vi "file_io_vi.vi"() -> ()   [LabVIEW 2017]
panel:
  out "letter count":dbl
  out "word count":dbl
  out "j":i32
  out "Array":string[](array[string])
  out "i":i32
  in  "delimiters":string[](array[string])
  out "result array":string[][](array[string])
  in  "format string":string
  in  "array type":string[][](array[string])
  out "text read from file":string
  out "error from read file":errorcluster
  in  "file path (read file)":path
  out "error from write file":errorcluster
  in  "text will be written to file":string
  in  "file path (write file)":path
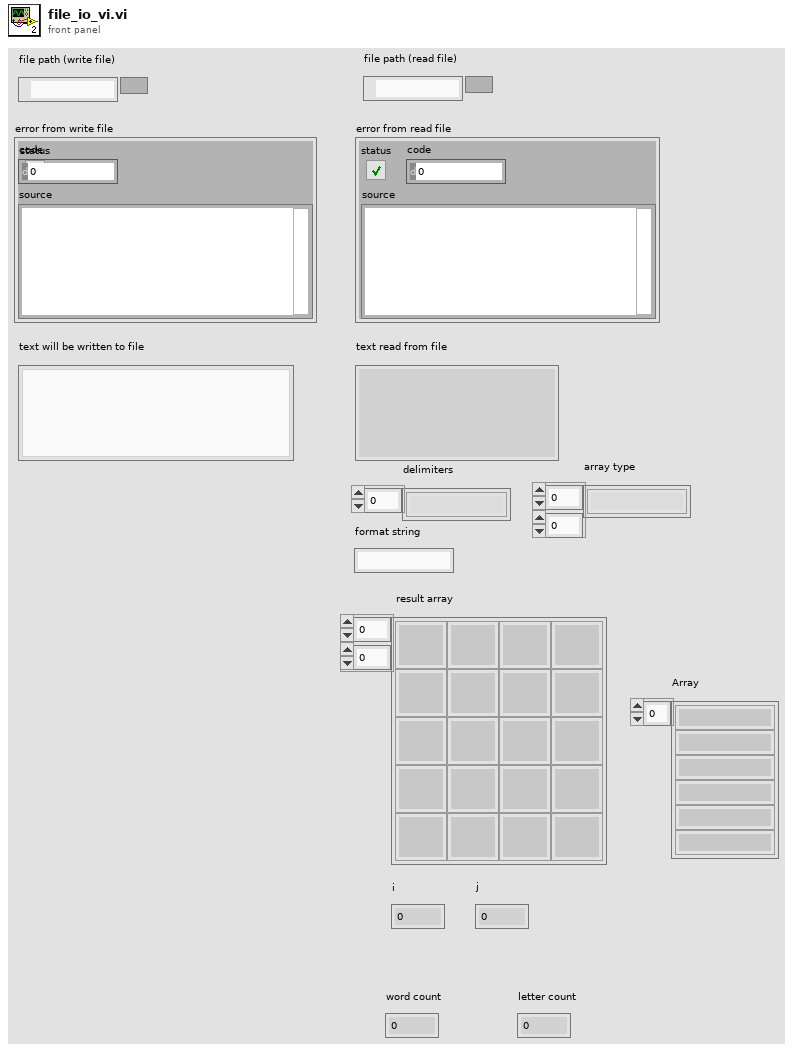
[diagram p1: front panel]
types:
  T1 = enum16{"open", "replace", "create", "open or create", "replace or create", "replace or create with confirmation"}
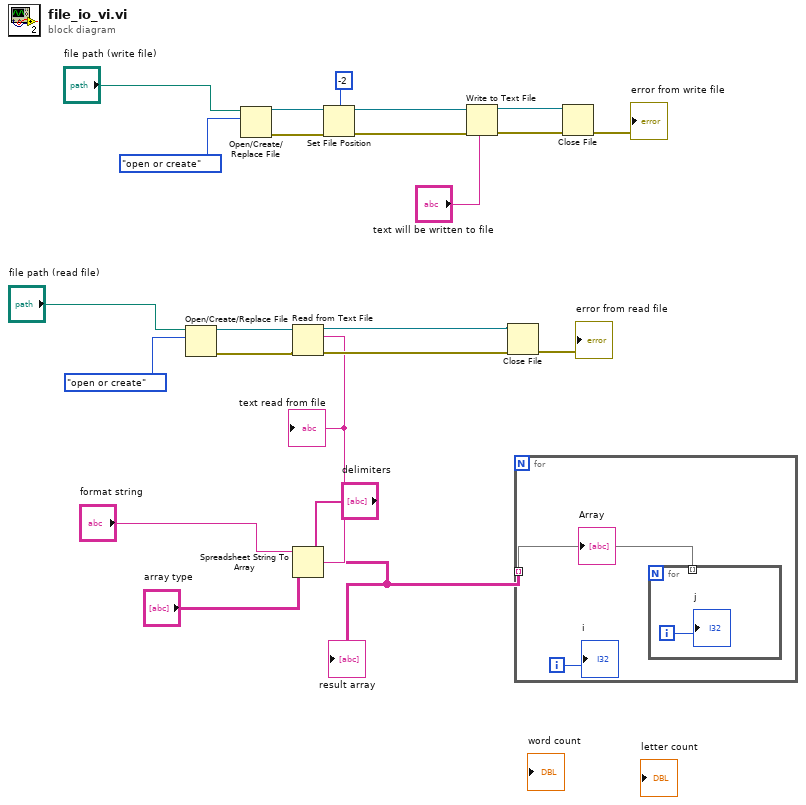
[diagram p0: block diagram]
diagram:
  n1 = Open/Create/Replace File(file path (use dialog)="file path (read file)", operation (0:open)=T1."open or create") -> (refnum out=w9:refnum<file>, error out=w7:errorcluster)  [unwired: 4 in, 1 out]
  n2 = Open/Create/Replace File(file path (use dialog)="file path (write file)", operation (0:open)=T1."open or create") -> (refnum out=w18:refnum<file>, error out=w15:errorcluster)  [unwired: 4 in, 1 out]
  n3 = Read from Text File(file (use dialog)=w9, error in=w7) -> (refnum out=w8:refnum<file>, text=w3:string, error out=w6:errorcluster)  [unwired: 2 in, 1 out]
  "text read from file" <- w3
  n4 = Spreadsheet String To Array(delimiter (Tab)="delimiters", format string="format string", spreadsheet string=w3, array type (2D Dbl)="array type") -> (array=w1:string[][])
  "result array" <- w1
  n5 = Set File Position(offset (in bytes) (0)=i64 -2, refnum=w18, error in=w15) -> (refnum out=w19:refnum<file>, error out=w14:errorcluster)  [unwired: 1 in]
  n6 = Write to Text File(file (use dialog)=w19, text="text will be written to file", error in=w14) -> (refnum out=w20:refnum<file>, error out=w13:errorcluster)  [unwired: 1 in, 1 out]
  n7 = Close File(refnum=w8, error in=w6) -> (error out=→"error from read file":errorcluster)  [unwired: 1 out]
  n8 = for {
    tunnel: w1 -> [w24] mode=indexing
    i -> [w25]
    n9 = for {
      tunnel: w24 -> [_] mode=indexing
      i -> [w26]
      "j" <- w26
    }
    "i" <- w25
    "Array" <- w24
  }
  n10 = Close File(refnum=w20, error in=w13) -> (error out=→"error from write file":errorcluster)  [unwired: 1 out]
